vi "Request Multiple Addresses.vi"(8 "error in (no error)":errorcluster, 11 "connection info":T3) -> (0 "error out":errorcluster, 2 "variant":variant, 3 "connection info":T3, 4 "Error Array":T1[](array[typedef]))   [LabVIEW 2019, in "J1939 Addon Shared.lvlib"]
uses:
  J1939 Addon Shared.lvlib
  <vilib>/NI/STM/TCP/TCP Connection Info.ctl
  <vilib>/NI/STM/SubVIs/MetaDataElement.ctl
  Types/Error Cluster.ctl
  Types/Error Types.ctl
  <vilib>/NI/STM/NI STM.lvlib
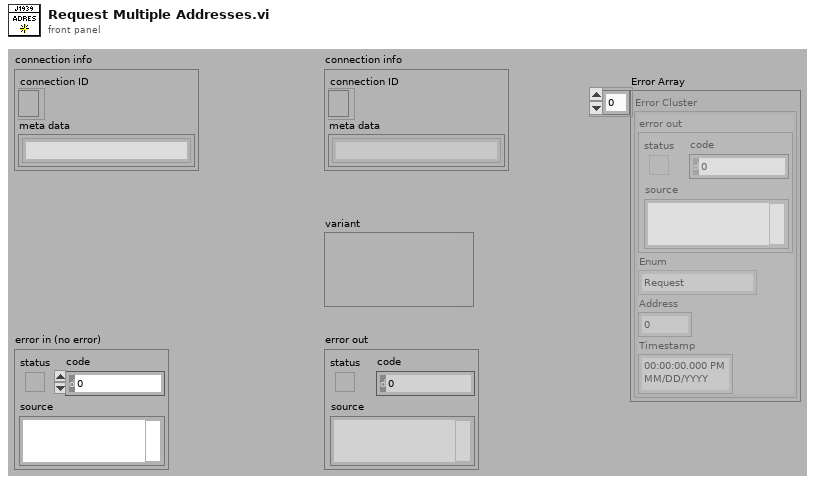
[diagram p1: front panel]
types:
  T1 = typedef "J1939 Addon Shared.lvlib/Error Cluster.ctl" = cluster{"error out":errorcluster, "Enum":T2, "Address":u8, "Timestamp":timestamp}
  T2 = typedef "J1939 Addon Shared.lvlib/Error Types.ctl" = enum16{"Request", "RAW Generation", "Clear Active DTCs", "Clear Previous DTCs", "Addresses", "TLAs", "Get Active DTCs", "Get Previous DTCs", "TCP Connection"}
  T3 = typedef "NI STM.lvlib/TCP Connection Info.ctl" = cluster{"connection ID":refnum<k5>, "meta data":T4[]}
  T4 = typedef "NI STM.lvlib/MetaDataElement.ctl" = string
  T5 = typedef "J1939 Addon Shared.lvlib/Address Lookup Table Data.ctl" = cluster{"Name":u8[], "Address":u8}
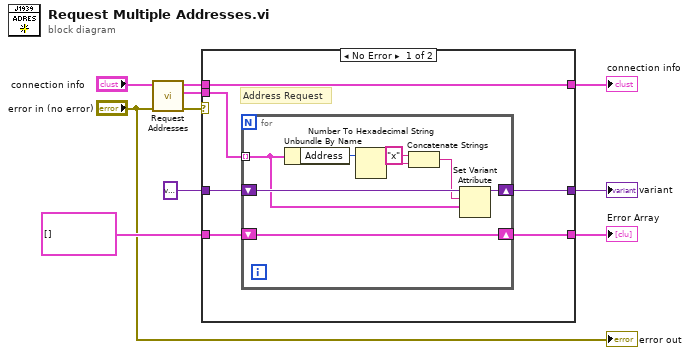
[diagram p0: block diagram]
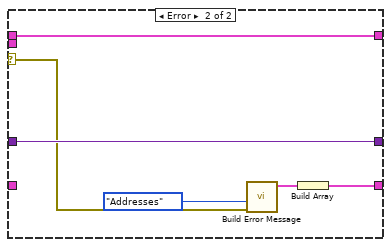
[diagram p2: hidden frame]
diagram:
  n1 = call "Request Addresses.vi"("error in (no error)"="error in (no error)", "connection info"="connection info") -> ("error out"=w1:errorcluster, "All Data"=w9:T5[], "connection info"=w10:T3)  [unwired: 7 in]
  n2 = case shown="No Error" w1 {
    selector: w1 -> [_ w28]
    tunnel: w10 -> [w11 w30]
    tunnel: w9 -> [w12 _]
    tunnel: [w16 w29] -> w8
    tunnel: [w11 w30] -> w7
    tunnel: variant ("variant") -> [w15 w29]
    tunnel: T1[] [] -> [w14 _]
    tunnel: [w13 w26] -> w3
    frame No Error {
      # "Address Request"
      n3 = for {
        shift-right: [w24] -> w16
        shift-left: w15 -> [w23]
        shift-right: [w22] -> w13
        shift-left: w14 -> [w22]
        tunnel: w12 -> [w21] mode=indexing
        n4 = Unbundle By Name(w21) -> ("Address"=w20:u8)
        n5 = Number To Hexadecimal String(2:w20) -> (0:w19:string)  [unwired: 1 in]
        n6 = Concatenate Strings("x" ("string"), w19) -> (w18:string)
        n7 = Set Variant Attribute(Variant=w23, name=w18, value=w21) -> (Variant out=w24:variant)  [unwired: 1 in, 2 out]
      }
    }
    frame Error {
      n8 = call "Build Error Message.vi"("error IO"=w28, "Enum"=Error_Types."Addresses") -> ("Error Cluster"=w27:T1)  [unwired: 9 in]
      n9 = Build Array(w27) -> (w26:T1[])
    }
  }
  "variant" <- w8
  "connection info" <- w7
  "Error Array" <- w3
  "error out" <- "error in (no error)"
